vi "수신.vi"() -> ()   [LabVIEW 2014]
panel:
  out "웨이브폼 그래프":dbl[](graph)
  in  "정지":bool
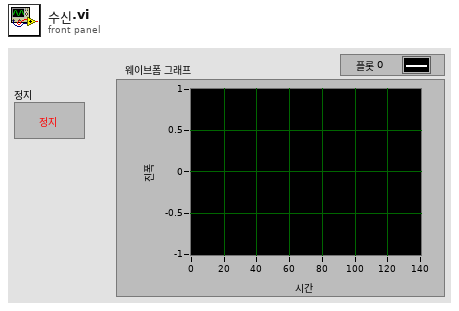
[diagram p1: front panel]
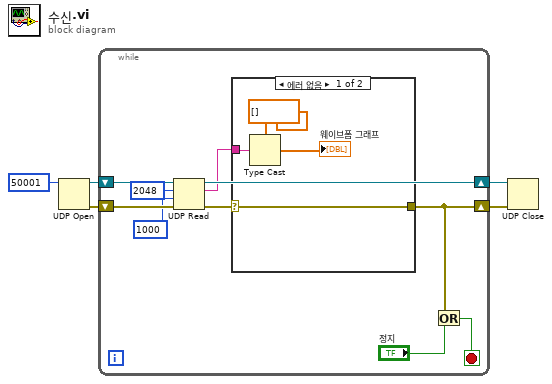
[diagram p0: block diagram]
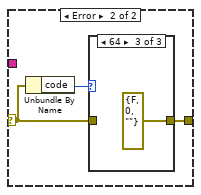
[diagram p2: hidden frame]
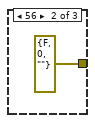
[diagram p4: hidden frame]
diagram:
  n1 = UDP Open(11:u16 50001 ("포트")) -> (port=w5:refnum<k16>, 0:w2:errorcluster)  [unwired: 4 in, 1 out]
  n2 = while {
    shift-right: [w14] -> w4
    shift-left: w5 -> [w15]
    shift-right: [w9] -> w1
    shift-left: w2 -> [w13]
    stop <- w10 stop-if-true
    n3 = UDP Read(connection ID=w15, max size (548)=2048 ("최대 크기(548)"), timeout ms (25000)=1000 ("타임아웃 ms (25000)"), 8:w13) -> (data out=w12:string, error out=w11:errorcluster, 3:w14:refnum<k16>)  [unwired: 2 out]
    n4 = case shown="에러 없음" w11 {
      selector: w11 -> [w19 w21]
      tunnel: w12 -> [w18 _]
      tunnel: [w19 w20] -> w9
      frame No Error {
        n5 = Type Cast(type=dbl[] [] ("웨이브폼 그래프"), x=w18) -> (*(type *) &x=→"웨이브폼 그래프":dbl[])
      }
      frame Error {
        n6 = Unbundle By Name(w21) -> ("code"=w22:i32)
        n7 = case shown="64" w22 {
          tunnel: w21 -> [w23 _ _]
          tunnel: [w23 errorcluster {"status"=FALSE, "code"=0, "source"=""} ("에러 상수") errorcluster {"status"=FALSE, "code"=0, "source"=""} ("에러 상수")] -> w20
          frame Default {
          }
          frame 56 {
          }
          frame 64 {
          }
        }
      }
    }
    n8 = Or(x=w9, y="정지") -> (x .or. y?=w10:bool)
  }
  n9 = UDP Close(connection ID=w4, 8:w1) -> ()  [unwired: 2 out]
